vi "GetWfgEnabled.vi"(0 "object in":refnum<class "InstrumentBase.lvclass">, 5 "error in (no error)":errorcluster) -> (14 "object out":refnum<class "InstrumentBase.lvclass">, 15 "WfgEnabled":cluster{"Ch1":bool, "Ch2":bool}, 19 "error out":errorcluster)   [LabVIEW 2019, in "InstrumentBase.lvclass"]
uses:
  InstrumentBase.lvclass
  InstrumentBase.lvclass/InstrumentBase.ctl
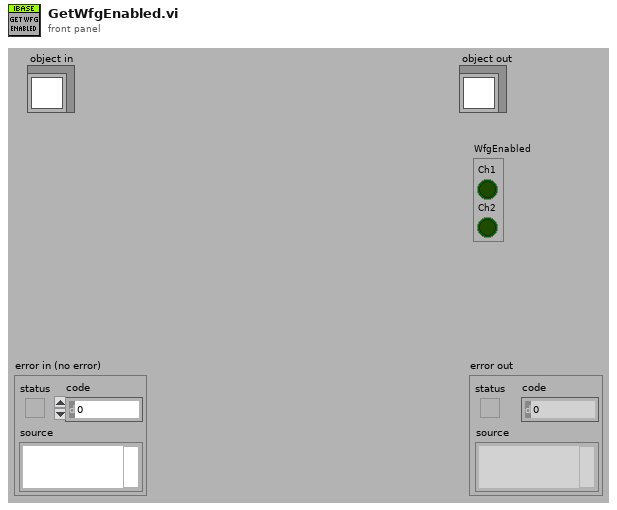
[diagram p1: front panel]
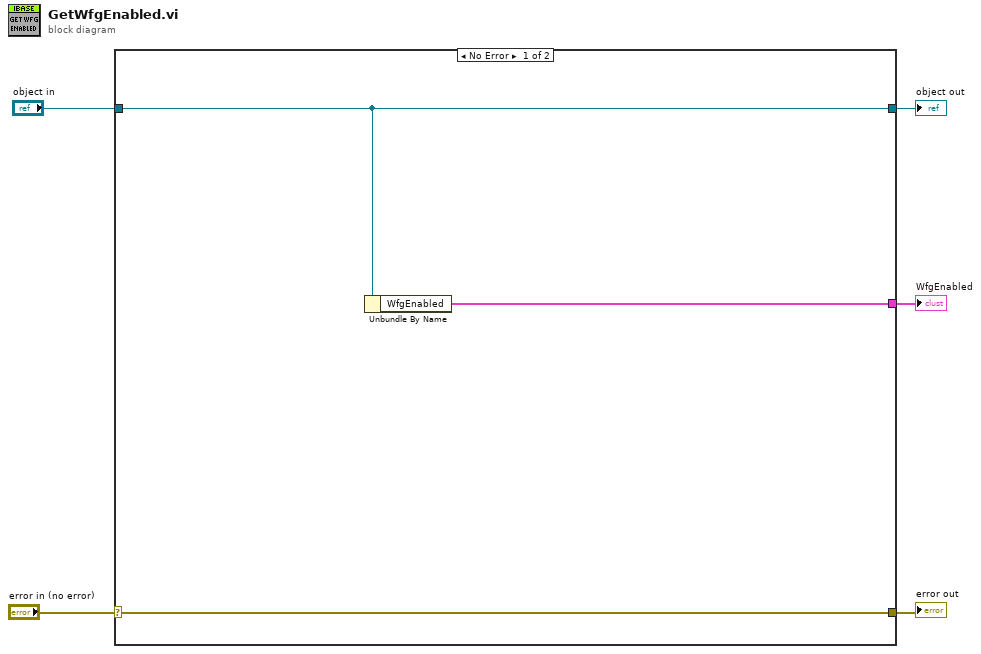
[diagram p0: block diagram]
diagram:
  n1 = case shown="No Error" "error in (no error)" {
    selector: "error in (no error)" -> [w7 w10]
    tunnel: [w7 w10] -> w4
    tunnel: [w6 w9] -> w2
    tunnel: "object in" -> [w6 w9]
    tunnel: [w8 _] -> w1
    frame No Error {
      n2 = Unbundle By Name(w6) -> ("WfgEnabled"=w8:cluster{"Ch1":bool, "Ch2":bool})
    }
    frame Error {
    }
  }
  "error out" <- w4
  "object out" <- w2
  "WfgEnabled" <- w1
